vi "NI_FPGA_PPG.publish device status.vi"(0 "i ref in":refnum<vi>, 2 "actual_status":i32, 3 "ms timeout (10000)":i32=10000, 5 "error in (no error)":errorcluster) -> (14 "i ref out":refnum<vi>, 17 "timed out":bool, 19 "error out":errorcluster)   [LabVIEW 2014, in "NI_FPGA_PPG.lvlib"]
doc: "Publishes the device status via DIM.\n\nLicense Agreement for this software:\n\nCopyright (C) 2009\nFalk Ziegler\nInstitut für Physik\nErnst-Moritz-Arndt Universität\nFelix-Hausdorff-Str. 6\n17487 Greifswald\n\nContact: Falk Ziegler, ziegler@physik.uni-greifswald.de\n\nThis program is free software: you can redistribute it and/or modify it under the terms of the GNU General Public License as published by the Free Software Foundation, either version 3 of the License, or (at your option) any later version.\n\nThis program is distributed in the hope that it will be useful, but WITHOUT ANY WARRANTY; without even the implied warranty of MERCHANTABILITY or FITNESS FOR A PARTICULAR PURPOSE. See the GNU General Public License for more details.\n\nYou should have received a copy of the GNU General Public License along with this program. If not, see <http://www.gnu.org/licenses/>.\n\nFor all questions and ideas contact: ziegler@physik.uni-greifswald.de or d.beck@gsi.de\nLast update: 01-Sep-2009"
uses:
  NI_FPGA_PPG.lvlib
  CSlibraries-extern/DimLVEvent/LVDimInterface/LVDimInterface.lvlib
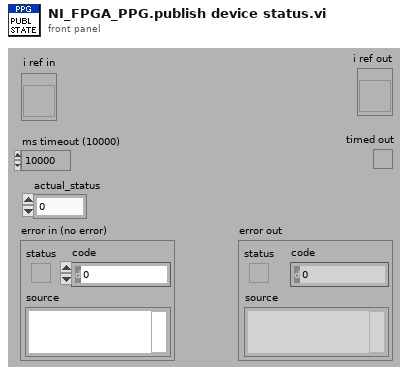
[diagram p1: front panel]
types:
  T1 = typedef "NI_FPGA_PPG.lvlib/NI_FPGA_PPG.i attribute.ctl" = cluster{"dim_service_id":cluster{"dim_actual_device_status":i32, "dim_event_data":i32, "dim_cmd_data":i32, "dim_cmd_data _description":i32, "dim_channel_description":i32}, "VISA":refnum<visa-resource-name>, "actual_device_status":i32, "event_data_id":i32, "pdc_enabled":bool, "pdc_timestamp":u32, "cmd_data_string":string, "cmd_data_size":i32, "cmd_data_description_string":string, "cmd_data_description_size":i32, "channel_description_string":string, "channel_description_size":i32}
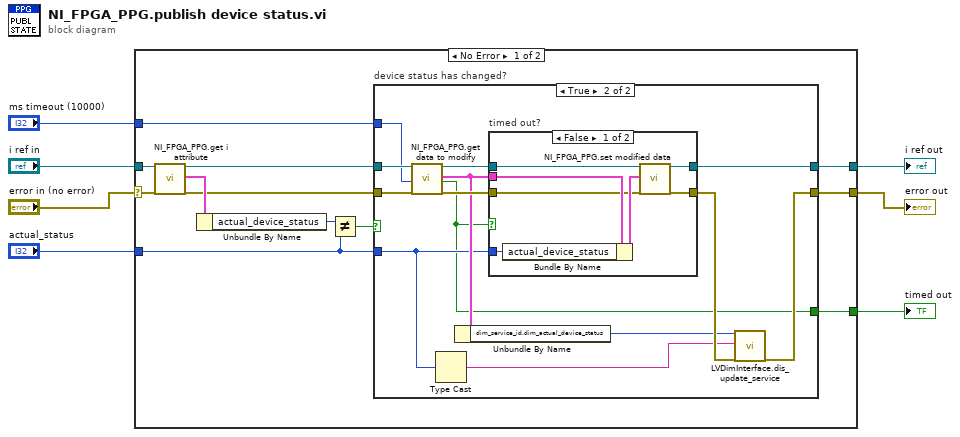
[diagram p0: block diagram]
diagram:
  n1 = case shown="No Error" "error in (no error)" {
    selector: "error in (no error)" -> [w11 w44]
    tunnel: "i ref in" -> [w12 w45]
    tunnel: [w14 w45] -> w5
    tunnel: [w13 w44] -> w4
    tunnel: "ms timeout (10000)" -> [w15 _]
    tunnel: "actual_status" -> [w9 _]
    tunnel: [w8 _] -> w1
    frame No Error {
      n2 = call "NI_FPGA_PPG.get i attribute.vi"("i ref in"=w12, "error in (no error)"=w11) -> ("i ref out"=w17:refnum<vi>, "i attribute"=w19:T1, "error out"=w16:errorcluster)  [unwired: 15 in]
      n3 = Unbundle By Name(w19) -> ("actual_device_status"=w10:i32)
      n4 = Not Equal?(x=w10, y=w9) -> (x != y?=w18:bool)
      n5 = case "device status has changed?" shown="True" w18 {
        tunnel: w17 -> [w21 w34]
        tunnel: w16 -> [w20 w32]
        tunnel: w15 -> [_ w33]
        tunnel: [w21 w29] -> w14
        tunnel: [w20 w26] -> w13
        tunnel: w9 -> [_ w24]
        tunnel: [_ w22] -> w8
        frame False {
        }
        frame True {
          n6 = call "NI_FPGA_PPG.get data to modify.vi"("i ref in"=w34, "ms timeout (10000)"=w33, "error in (no error)"=w32) -> ("i ref out"=w31:refnum<vi>, "i attribute"=w28:T1, "timed out"=w22:bool, "error out"=w30:errorcluster)  [unwired: 13 in]
          n7 = Type Cast(x=w24) -> (*(type *) &x=w23:string)  [unwired: 1 in]
          n8 = Unbundle By Name(w28) -> ("dim_service_id.dim_actual_device_status"=w25:i32)
          n9 = case "timed out?" shown="False" w22 {
            tunnel: w31 -> [w36 w43]
            tunnel: w30 -> [w37 w42]
            tunnel: w28 -> [w39 _]
            tunnel: [w41 w43] -> w29
            tunnel: [w40 w42] -> w27
            tunnel: w24 -> [w35 _]
            frame False {
              n10 = Bundle By Name(cluster=w39, "actual_device_status"=w35) -> (w38:T1)
              n11 = call "NI_FPGA_PPG.set modified data.vi"("i ref in"=w36, "i attribute"=w38, "error in (no error)"=w37) -> ("i ref out"=w41:refnum<vi>, "error out"=w40:errorcluster)  [unwired: 15 in]
            }
            frame True {
            }
          }
          n12 = call "LVDimInterface.dis_update_service.vi"("my_serviceID"=w25, "data"=w23, "error in (no error)"=w27) -> ("error out"=w26:errorcluster)  [unwired: 14 in, 2 out]
        }
      }
    }
    frame Error {
    }
  }
  "error out" <- w4
  "i ref out" <- w5
  "timed out" <- w1
